vi "Sonar.vi"() -> ()   [LabVIEW 2020]
uses:
  <vilib>/MakerHub/LINX/Public/Utilities/Open Serial.vi
  <vilib>/MakerHub/LINX/Public/Sensors/Motion/Servo/Servo Open One Channel.vi
  <vilib>/MakerHub/LINX/Public/Sensors/Motion/Servo/Servo Close One Channel.vi
  <vilib>/MakerHub/LINX/LMH-LINX.lvlib
  <vilib>/MakerHub/LINX/Public/Sensors/Motion/Servo/Servo.lvlib
panel:
  out "Sonar":picture
  out "Distance":dbl
  out "Warning":string="Input Too High"
  out "Turning Angle":dbl
  in  "stop":bool
  in  "Servo Channel":u8
  in  "Trigger Pin":u8
  in  "Echo Pin":u8
  in  "Serial Port":refnum<visa-resource-name>="N/A"
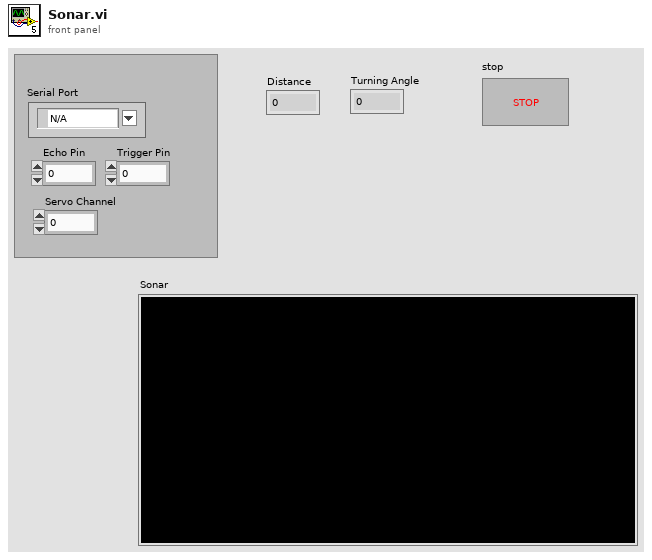
[diagram p1: front panel]
types:
  T1 = typedef "LMH-LINX.lvlib/LINX Ref.ctl" = cluster{"IO":T2, "Interface":T3, "LINX Device Config":T4}
  T2 = typedef "LMH-LINX.lvlib/Platform.ctl" = enum16{"Remote", "Local"}
  T3 = typedef "LMH-LINX.lvlib/Interface.ctl" = enum16{"Serial", "TCP"}
  T4 = typedef "LMH-LINX.lvlib/Device.lvlib/LINX Device Config.ctl" = cluster{"Interface":T3, "COM Port":refnum<visa-resource-name>, "TCP Configuration":T5, "Device Family":u8, "Device ID":u8, "Device Name":string, "TCP Ref":refnum<k5>, "Channels":T6}
  T5 = typedef "LMH-LINX.lvlib/Device.lvlib/TCP Config.ctl" = cluster{"IP Address":string, "Port":u16}
  T6 = typedef "LMH-LINX.lvlib/Channels.ctl" = cluster{"DI":u8[], "DO":u8[], "AI":u8[], "AO":u8[], "PWM":u8[], "QE":u8[], "UART":u8[], "I2C 2":u8[], "SPI":u8[], "CAN":u8[], "Servo":u8[], "AI Ref (V)":dbl, "AI Resolution (Bits)":u8, "AO Ref (V)":dbl, "AO Resolution (Bits)":u8}
  T7 = cluster{"maximum":dbl, "minimum":dbl, "clip to min":bool, "log?(F)":bool, "grid color":u32, "plot color":u32, "fmt and prec":cluster{"format":enum8{"Decimal", "Scientific", "Engineering", "Binary", "Octal", "Hex"}, "precision":u8}, "visible section":u16}
  T8 = typedef "imagedata.ctl" = cluster{"image type":i32, "image depth":i32, "image":u8[], "mask":u8[], "colors":u32[], "Rectangle":cluster{"left":i16, "top":i16, "right":i16, "bottom":i16}}
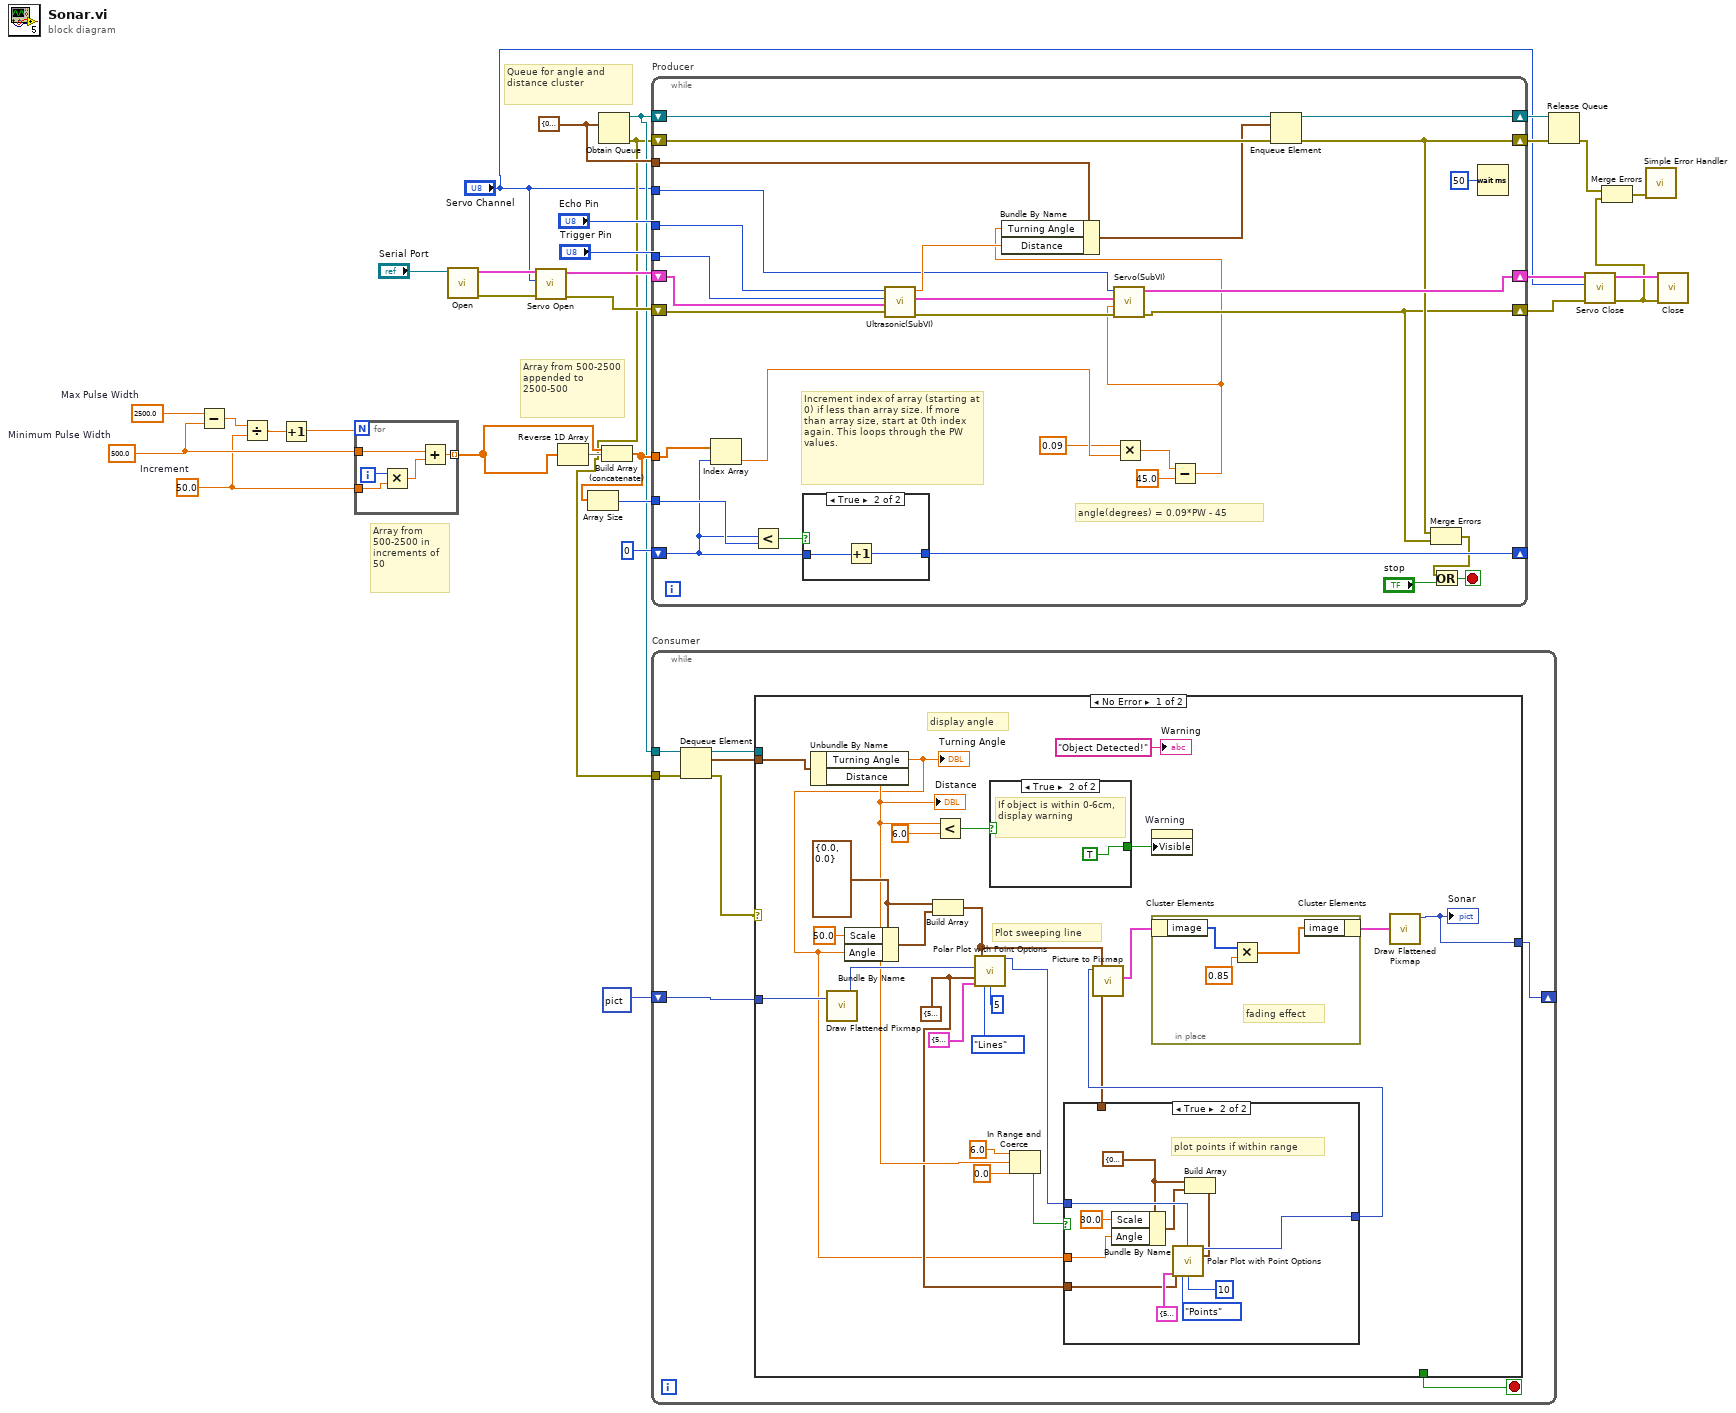
[diagram p0: block diagram]
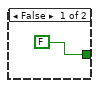
[diagram p3: hidden frame]
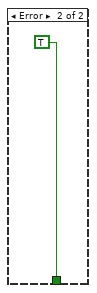
[diagram p4: hidden frame]
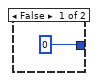
[diagram p5: hidden frame]
diagram:
  w10 = cluster{"Turning Angle":dbl, "Distance":dbl} {"Turning Angle"=0.0, "Distance"=0.0}
  w30 = 50.0  # Increment
  w31 = 500.0  # Minimum Pulse Width
  w28 = 2500.0  # Max Pulse Width
  # "Queue for angle and distance cluster"
  # "Array from 500-2500 appended to 2500-500"
  # "Array from 500-2500 in increments of 50"
  n1 = Subtract(x=w28, y=w31) -> (x-y=w26:dbl)
  n2 = Divide(x=w26, y=w30) -> (x/y=w27:dbl)
  n3 = Increment(x=w27) -> (x+1=w29:dbl)
  n4 = for {
    N: w29 -> [_]
    tunnel: w30 -> [w34]
    tunnel: w31 -> [w33]
    tunnel: [w32] -> w22 mode=indexing
    i -> [w35]
    n5 = Multiply(x=w35, y=w34) -> (x*y=w36:dbl)
    n6 = Add(x=w33, y=w36) -> (x+y=w32:dbl)
  }
  n7 = call-poly <vilib>:"Open.vi"("Serial Port"="Serial Port") -> ("Error Out"=w17:errorcluster, "LINX Resource"=w19:T1)  [unwired: 8 in, 1 out]
  n8 = call-poly <vilib>:"Servo Open.vi"("Error In"=w17, "Servo Channel"="Servo Channel", "LINX Resource"=w19) -> ("Error Out"=w16:errorcluster, "LINX Resource"=w18:T1)  [unwired: 7 in]
  n9 = Reverse 1D Array(array=w22) -> (reversed array=w23:dbl[])
  n10 = Obtain Queue(element data type=w10) -> (queue out=w4:refnum<queue>, error out=w3:errorcluster)  [unwired: 4 in, 1 out]
  n11 = Build Array (concatenate)(w22, w23) -> (w21:dbl[])
  n12 = Array Size(array=w21) -> (size(s)=w24:i32)
  n13 = while "Producer" {
    tunnel: w24 -> [w65]
    shift-right: [w63] -> _
    shift-left: 0 -> [w64]
    tunnel: w21 -> [w62]
    tunnel: "Echo Pin" -> [w57]
    tunnel: "Trigger Pin" -> [w56]
    tunnel: "Servo Channel" -> [w38]
    shift-right: [w47] -> w14
    shift-left: w16 -> [w59]
    shift-right: [w55] -> w15
    shift-left: w18 -> [w61]
    tunnel: w10 -> [w52]
    shift-right: [w49] -> w8
    shift-left: w4 -> [w54]
    shift-right: [w48] -> w9
    shift-left: w3 -> [w53]
    stop <- w46 stop-if-true
    # "angle(degrees) = 0.09*PW - 45"
    # "Increment index of array (starting at 0) if less than array size. If more than array size, start at 0th index again. This loops through the PW values."
    n14 = Index Array(array=w62, index=w64) -> (element=w43:dbl)
    n15 = Less?(x=w64, y=w65) -> (x < y?=w66:bool)
    n16 = case shown="True" w66 {
      tunnel: w64 -> [_ w69]
      tunnel: [0 w68] -> w63
      frame False {
      }
      frame True {
        n17 = Increment(x=w69) -> (x+1=w68:i32)
      }
    }
    n18 = call "Ultrasonic(SubVI).vi"("error in (no error)"=w59, "LINX Resource in"=w61, "Trigger Pin"=w56, "Echo Pin"=w57) -> ("error out"=w58:errorcluster, "LINX Resource out"=w60:T1, "Centimeters"=w51:dbl)  [unwired: 4 in, 1 out]
    n19 = Multiply(x=0.09, y=w43) -> (x*y=w41:dbl)
    n20 = Subtract(x=w41, y=45.0) -> (x-y=w37:dbl)
    n21 = Bundle By Name(cluster=w52, "Turning Angle"=w37, "Distance"=w51) -> (w50:cluster{"Turning Angle":dbl, "Distance":dbl})
    n22 = call "Servo(SubVI).vi"("error in (no error)"=w58, "Position"=w37, "LINX Resource in"=w60, "Servo Channel"=w38) -> ("error out"=w47:errorcluster, "LINX Resource out"=w55:T1)  [unwired: 6 in]
    n23 = Enqueue Element(queue=w54, element=w50, error in (no error)=w53) -> (queue out=w49:refnum<queue>, error out=w48:errorcluster)  [unwired: 1 in, 1 out]
    n24 = Merge Errors(w48, w47) -> (w45:errorcluster)
    n25 = Or(x=w45, y="stop") -> (x .or. y?=w46:bool)
    n26 = Wait (ms)(milliseconds to wait=u32 50) -> ()  [unwired: 1 out]
  }
  n27 = while "Consumer" {
    tunnel: w4 -> [w77]
    tunnel: w3 -> [w73]
    shift-right: [w70] -> _
    shift-left: picture data[5B] ("picture") -> [w71]
    stop <- w72 stop-if-true
    n28 = Dequeue Element(queue=w77, error in (no error)=w73) -> (queue out=w74:refnum<queue>, element=w75:cluster{"Turning Angle":dbl, "Distance":dbl}, error out=w76:errorcluster)  [unwired: 1 in, 1 out]
    n29 = case shown="No Error" w76 {
      tunnel: w75 -> [w81 _]
      tunnel: w74 -> [_ _]
      tunnel: [_ TRUE] -> w72
      tunnel: w71 -> [w96 _]
      tunnel: [w89 _] -> w70
      frame No Error {
        w94 = cluster{"Scale":dbl, "Angle":dbl} {"Scale"=0.0, "Angle"=0.0}
        w79 = cluster{"width":i16, "height":i16} {"width"=500, "height"=0} ("dimensions (w,h)")
        # "Plot sweeping line"
        # "display angle"
        n30 = Unbundle By Name(w81) -> ("Turning Angle"=w78:dbl, "Distance"=w85:dbl)
        "Turning Angle" <- w78
        "Distance" <- w85
        n31 = call <vilib>:"Draw Flattened Pixmap.vi"("picture"=w96) -> ("new picture"=w95:picture)  [unwired: 8 in]
        n32 = Bundle By Name(cluster=w94, "Scale"=50.0, "Angle"=w78) -> (w93:cluster{"Scale":dbl, "Angle":dbl})
        n33 = Build Array(w94, w93) -> (w80:cluster{"Scale":dbl, "Angle":dbl}[])
        n34 = Less?(x=w85, y=6.0) -> (x < y?=w101:bool)
        n35 = call <vilib>:"Polar Plot with Point Options.vi"("picture"=w95, "data array [mag, phase (deg)]"=w80, "dimensions (w,h)"=w79, "polar attributes"=T7 {"maximum"=50.0, "minimum"=10.0, "clip to min"=TRUE, "log?(F)"=FALSE, "grid color"=6710886, "plot color"=2621184, "fmt and prec"={"format"=enum."Decimal", "precision"=0}, "visible section"=4}, "Lines/Points"=enum16{"Lines", "Points"}."Lines", "Size"=u16 5) -> ("new picture"=w83:picture)  [unwired: 9 in]
        n36 = case shown="True" w101 {
          tunnel: [FALSE ("Visible") TRUE ("Visible")] -> w99
          frame False {
          }
          frame True {
            # "If object is within 0-6cm, display warning"
          }
        }
        n37 = In Range and Coerce(upper limit=6.0, x=w85, lower limit=0.0) -> (In Range?=w84:bool)  [unwired: 1 out]
        n38 = case shown="True" w84 {
          tunnel: w83 -> [w103 w114]
          tunnel: [w103 w113] -> w82
          tunnel: w80 -> [_ _]
          tunnel: w79 -> [_ w110]
          tunnel: w78 -> [_ w104]
          frame False {
          }
          frame True {
            w108 = cluster{"Scale":dbl, "Angle":dbl} {"Scale"=0.0, "Angle"=0.0}
            # "plot points if within range"
            n39 = Bundle By Name(cluster=w108, "Scale"=30.0, "Angle"=w104) -> (w107:cluster{"Scale":dbl, "Angle":dbl})
            n40 = Build Array(w108, w107) -> (w105:cluster{"Scale":dbl, "Angle":dbl}[])
            n41 = call <vilib>:"Polar Plot with Point Options.vi"("picture"=w114, "data array [mag, phase (deg)]"=w105, "dimensions (w,h)"=w110, "polar attributes"=T7 {"maximum"=50.0, "minimum"=10.0, "clip to min"=TRUE, "log?(F)"=FALSE, "grid color"=6710886, "plot color"=16724242, "fmt and prec"={"format"=enum."Decimal", "precision"=0}, "visible section"=4}, "Lines/Points"=enum16{"Lines", "Points"}."Points", "Size"=u16 10) -> ("new picture"=w113:picture)  [unwired: 9 in]
          }
        }
        n42 = call <vilib>:"Picture to Pixmap.vi"("picture"=w82) -> ("image data"=w91:T8)  [unwired: 9 in, 1 out]
        n43 = property on="Warning" class="Str"("Visible"=w99) -> ()  [unwired: 2 in, 2 out]
        n44 = in-place {
          # "fading effect"
          n45 = in-place-cluster #1(w91) -> ("image"=w117:u8[])
          n46 = Multiply(x=w117, y=0.85) -> (x*y=w115:dbl[])
          n47 = in-place-cluster #1("image"=w115) -> (w90:T8)
        }
        n48 = call <vilib>:"Draw Flattened Pixmap.vi"("image data"=w90) -> ("new picture"=w89:picture)  [unwired: 8 in]
        "Sonar" <- w89
        "Warning" <- "Object Detected!" ("Warning")
      }
      frame Error {
      }
    }
  }
  n49 = Release Queue(queue=w8, error in (no error)=w9) -> (error out=w7:errorcluster)  [unwired: 1 in, 2 out]
  n50 = call-poly <vilib>:"Servo Close.vi"("Error In"=w14, "Servo Channel"="Servo Channel", "LINX Resource"=w15) -> ("Error Out"=w6:errorcluster, "LINX Resource"=w13:T1)  [unwired: 7 in]
  n51 = Merge Errors(w7, w6) -> (w5:errorcluster)
  n52 = call <vilib>:"Simple Error Handler.vi"("error in (no error)"=w5) -> ()  [unwired: 4 in, 5 out]
  n53 = call <vilib>:"Close.vi"("Error In"=w6, "LINX Resource"=w13) -> ()  [unwired: 9 in, 1 out]
